vi "DAQmxTaskContainerRelayKeyHeater-Com-Exec.vi"(8 "error in (no error)":errorcluster, 9 "ControlQueue":refnum<queue>, 10 "data":variant, 11 "DAQmxTaksContainer_General in":refnum<class "DAQmxTaksContainer_General.lvclass">) -> (0 "error out":errorcluster, 3 "DAQmxTaksContainer_General out":refnum<class "DAQmxTaksContainer_General.lvclass">)   [LabVIEW 2015, in "DAQmxTaksContainer_General.lvclass"]
uses:
  DAQmxTaksContainer_General.lvclass
  dependecies/ControlsVIs/Clusters-def/SERVER-Commands.ctl
  dependecies/ControlsVIs/Clusters-def/ProtypeCommand-DAQmxReply.ctl
  DAQmxTask.lvclass
  Control/Control-Server/Control-Server.lvclass
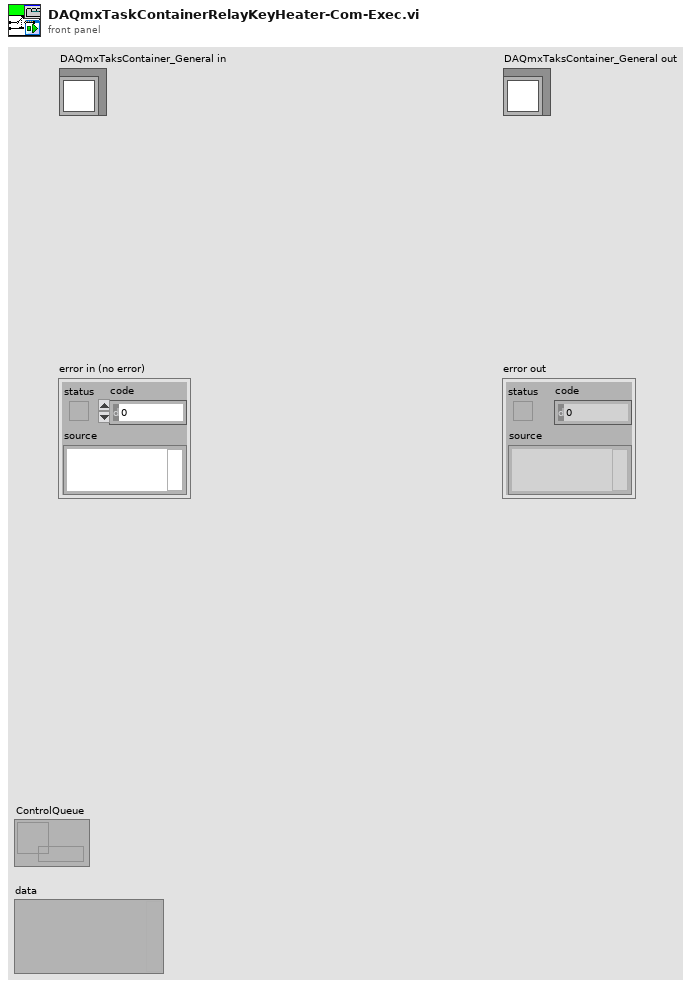
[diagram p1: front panel]
types:
  T1 = typedef "ProtypeCommand-DAQmxReply.ctl" = cluster{"On/Off":bool, "error out":errorcluster}
  T2 = typedef "Control-Server.lvclass/SERVER-Commands.ctl" = string
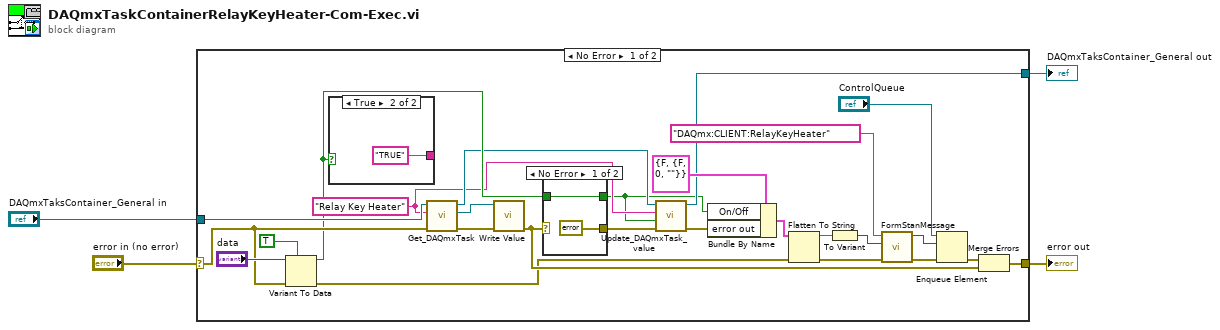
[diagram p0: block diagram]
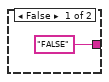
[diagram p2: hidden frame]
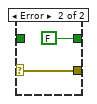
[diagram p3: hidden frame]
diagram:
  n1 = case shown="No Error" "error in (no error)" {
    selector: "error in (no error)" -> [w26 w38]
    tunnel: [w7 w37] -> w3
    tunnel: "DAQmxTaksContainer_General in" -> [w29 w37]
    tunnel: [w28 w38] -> w4
    frame No Error {
      w6 = "Relay Key Heater" ("Task name")
      n2 = Variant To Data(error in=w26, type=TRUE, Variant="data") -> (data=w20:bool, error out=w17:errorcluster)
      n3 = case shown="True" w20 {
        tunnel: ["FALSE" ("Data") "TRUE" ("Data")] -> _
        frame False {
        }
        frame True {
        }
      }
      n4 = call "Get_DAQmxTask.vi"("error in (no error)"=w26, "Task name"=w6, "DAQmxTaksContainer_General in"=w29) -> ("error out"=w25:errorcluster, "DAQmx Task"=w23:refnum<class "DAQmxTask.lvclass">, "DAQmxTaksContainer_General out"=w10:refnum<class "DAQmxTaksContainer_General.lvclass">)  [unwired: 6 in]
      n5 = call-dynamic "Write Value.vi"("error in (no error)"=w25, "DAQmxTask en entrée"=w23) -> ("error out"=w22:errorcluster)  [unwired: 8 in, 1 out]
      n6 = case shown="No Error" w22 {
        selector: w22 -> [_ w36]
        tunnel: [errorcluster {"status"=FALSE, "code"=5001, "source"="Relay key heater worked"} ("error constant") w36] -> w9
        tunnel: [w33 FALSE] -> w5
        tunnel: w20 -> [w33 _]
        frame No Error {
        }
        frame Error {
        }
      }
      n7 = call "Update_DAQmxTask_value.vi"("error in (no error)"=w9, "Value"=w5, "Task name"=w6, "DAQmxTaksContainer_General in"=w10) -> ("error out"=w8:errorcluster, "DAQmxTaksContainer_General out"=w7:refnum<class "DAQmxTaksContainer_General.lvclass">)  [unwired: 6 in]
      n8 = Bundle By Name(cluster=T1 {"On/Off"=FALSE, "error out"={"status"=FALSE, "code"=0, "source"=""}} ("output cluster"), "On/Off"=w5, "error out"=w8) -> (w18:T1)
      n9 = Flatten To String(anything=w18, error in (no error)=w17) -> (data string=w19:string, error out=w13:errorcluster)  [unwired: 2 in, 1 out]
      n10 = To Variant(anything=w19) -> (Variant=w14:variant)
      n11 = call "FormStanMessage.vi"("error in"=w13, "data"=w14, "Command"=T2 "DAQmx:CLIENT:RelayKeyHeater" ("command")) -> ("error out"=w12:errorcluster, "message"=w11:variant)  [unwired: 7 in]
      n12 = Enqueue Element(queue="ControlQueue", element=w11, error in (no error)=w12) -> (error out=w16:errorcluster)  [unwired: 1 in, 2 out]
      n13 = Merge Errors(w16, w22) -> (w28:errorcluster)
    }
    frame Error {
    }
  }
  "error out" <- w4
  "DAQmxTaksContainer_General out" <- w3
